vi "Filter String_Focus Handler_ACAF.vi"(5 "Disable":bool, 6 "Text Colors":T1, 7 "Make key focus?":bool, 8 "error in (no error)":errorcluster, 10 "Default Value":string, 11 "Filter String Ref":refnum<vi>) -> (0 "error out":errorcluster)   [LabVIEW 2023]
doc: "Call the filter and tree arrow handler. \n\nDown arrow or tab from filter goes to tree's first selectable item. Up arrow from filter goes to tree's last selectable item\n\nFilter arrows cycle on tree elements. Shift-tab from tree goes to filter"
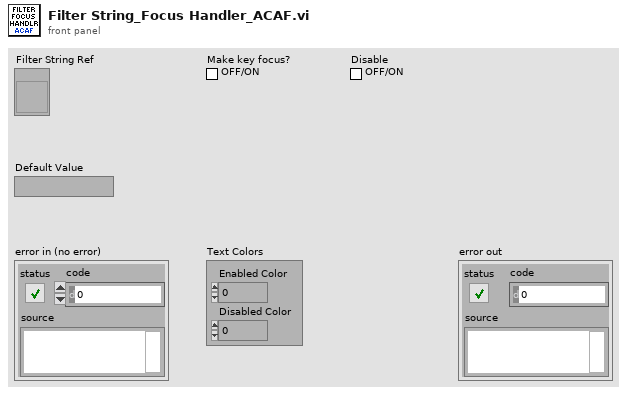
[diagram p1: front panel]
types:
  T1 = cluster{"Enabled Color":u32, "Disabled Color":u32}
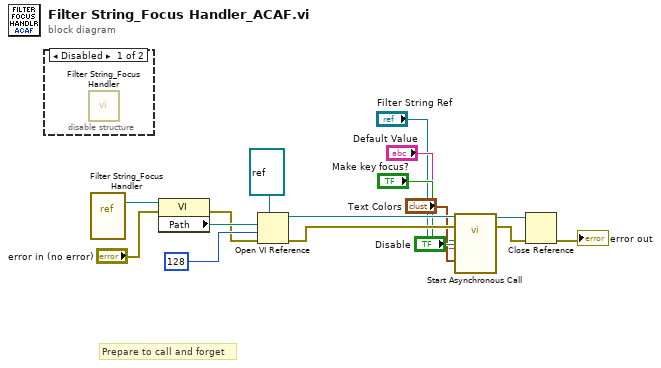
[diagram p0: block diagram]
diagram:
  # "Prepare to call and forget"
  n1 = disable-structure shown="Disabled" {
    frame Disabled {
      n2 = call "Filter String_Focus Handler.vi"() -> ()  [unwired: 12 in]
    }
    frame Enabled {
    }
  }
  n3 = vi-ref "Filter String_Focus Handler.vi"() -> (w16:refnum<vi>)
  n4 = property class="VI"(reference=w16, error in="error in (no error)") -> (error out=w6:errorcluster, "Path"=w12:path)  [unwired: 1 out]
  n5 = Open VI Reference(type specifier VI Refnum (for type only)=refnum<vi> refnum, vi path=w12, options=128, error in (no error)=w6) -> (vi reference=w7:refnum<vi>, error out=w11:errorcluster)  [unwired: 2 in]
  n6 = call-by-ref "Start Asynchronous Call"(reference=w7, error in=w11, "Disable"="Disable", "Text Colors"="Text Colors", "Make key focus?"="Make key focus?", "Default Value"="Default Value", "Filter String Ref"="Filter String Ref") -> (reference out=w10:refnum<vi>, error out=w9:errorcluster)  [unwired: 7 in]
  n7 = Close Reference(reference=w10, error in (no error)=w9) -> (error out=→"error out":errorcluster)
